vi "Update_Time.vi"(8 "error in (no error)":errorcluster, 9 "Reset?":bool, 10 "Advance?":bool, 11 "Elapsed Time In":dbl) -> (0 "error out":errorcluster, 2 "Display Out":string, 3 "Elapsed Time Out":dbl)   [LabVIEW 2026]
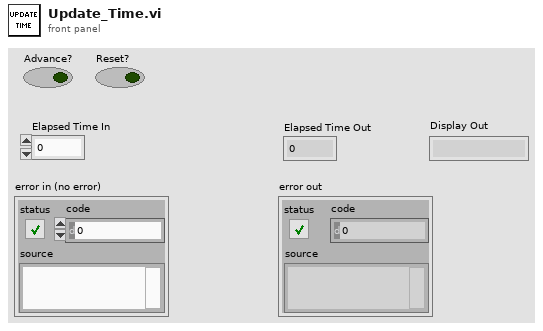
[diagram p1: front panel]
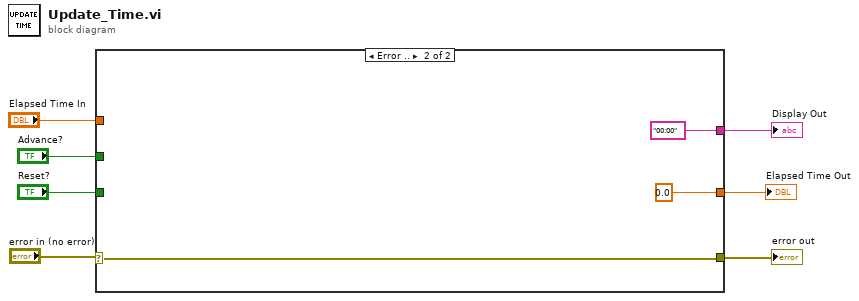
[diagram p0: block diagram]
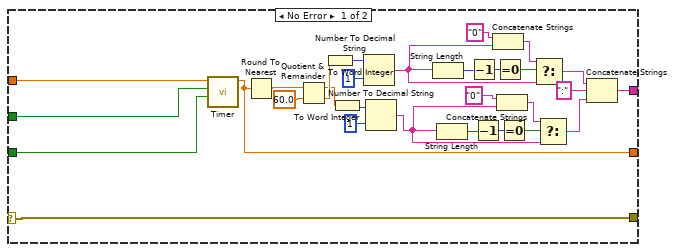
[diagram p2: hidden frame]
diagram:
  n1 = case shown="Error .." "error in (no error)" {
    selector: "error in (no error)" -> [w34 w39]
    tunnel: "Advance?" -> [w36 _]
    tunnel: "Reset?" -> [w35 _]
    tunnel: [w34 w39] -> w4
    tunnel: [w32 0.0 ("Elapsed Time Out")] -> w3
    tunnel: "Elapsed Time In" -> [w33 _]
    tunnel: [w29 "00:00"] -> w1
    frame No Error {
      n2 = call "Timer.vi"("Reset?"=w35, "Advance?"=w36, "Elapsed Time In"=w33) -> ("Elapsed Time Out"=w32:dbl)  [unwired: 8 in]
      n3 = Round To Nearest(number=w32) -> (nearest integer value=w28:dbl)
      n4 = Quotient & Remainder(x=w28, y=60.0) -> (x-y*floor(x/y)=w24:dbl, floor(x/y)=w26:dbl)
      n5 = To Word Integer(number=w26) -> (16bit integer=w25:i16)
      n6 = To Word Integer(number=w24) -> (16bit integer=w23:i16)
      n7 = Number To Decimal String(number=w25, width (-)=i16 1 ("precision (6)")) -> (decimal integer string=w16:string)
      n8 = Number To Decimal String(number=w23, width (-)=i16 1) -> (decimal integer string=w10:string)
      n9 = String Length(string=w16) -> (length=w20:i32)
      n10 = String Length(string=w10) -> (length=w13:i32)
      n11 = Decrement(x=w20) -> (x-1=w21:i32)
      n12 = Decrement(x=w13) -> (x-1=w14:i32)
      n13 = Concatenate Strings("0" ("string"), w16) -> (w17:string)
      n14 = Equal To 0?(x=w21) -> (x = 0?=w19:bool)
      n15 = Concatenate Strings("0" ("string"), w10) -> (w11:string)
      n16 = Equal To 0?(x=w14) -> (x = 0?=w12:bool)
      n17 = Select(t=w17, s=w19, f=w16) -> (s? t:f=w15:string)
      n18 = Select(t=w11, s=w12, f=w10) -> (s? t:f=w8:string)
      n19 = Concatenate Strings(w15, ":" ("string"), w8) -> (w29:string)
    }
    frame Error {
    }
  }
  "error out" <- w4
  "Elapsed Time Out" <- w3
  "Display Out" <- w1
